vi "Set Digital IO Mode.vi"(6 "Digital IO Mode (0: IN)":enum16{"Input", "Output", "Open Drain", ""}(ring), 8 "error in (no error)":errorcluster, 9 "Digital IO Trigger Type (0: Digital)":enum16{"Digital", "Trigger"}(ring), 10 "Digital IO Line (1)":u32=1, 11 "VISA resource name":refnum<visa-resource-name>) -> (0 "error out":errorcluster, 3 "VISA resource name out":refnum<visa-resource-name>)   [LabVIEW 2020, in "Keithley 2450.lvlib"]
doc: "Sets the digital I/O line to be a digital line or trigger model line and sets the line as an input or output. You can also use this VI to configure synchronous triggering modes."
uses:
  <instrlib>/Keithley 2450/Keithley 2450.lvlib
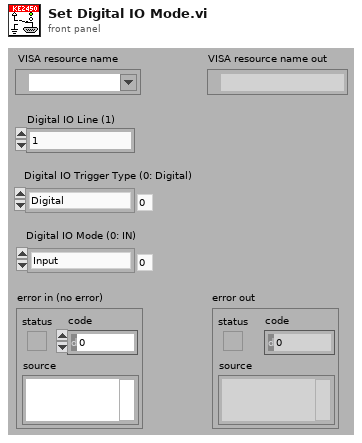
[diagram p1: front panel]
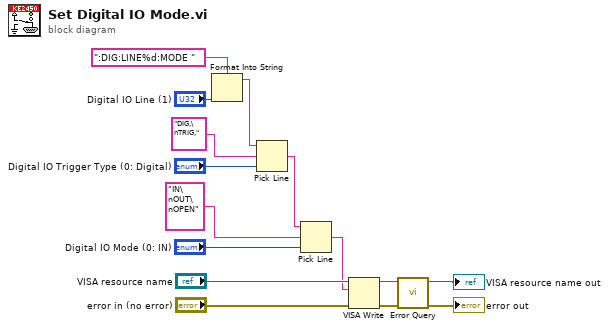
[diagram p0: block diagram]
diagram:
  n1 = Format Into String(format string=":DIG:LINE%d:MODE ", "Digital IO Line (1)") -> (resulting string=w6:string)  [unwired: 2 in, 1 out]
  n2 = Pick Line(string ("")=w6, multi-line string="DIG,\nTRIG,", line index="Digital IO Trigger Type (0: Digital)") -> (output string=w2:string)
  n3 = Pick Line(string ("")=w2, multi-line string="IN\nOUT\nOPEN", line index="Digital IO Mode (0: IN)") -> (output string=w1:string)
  n4 = VISA Write(VISA resource name="VISA resource name", write buffer=w1, error in (no error)="error in (no error)") -> (VISA resource name out=w13:refnum<visa-resource-name>, error out=w10:errorcluster)  [unwired: 1 out]
  n5 = call <instrlib>:"Error Query.vi"("error in (no error)"=w10, "VISA resource name"=w13) -> ("error out"=→"error out":errorcluster, "VISA resource name out"=→"VISA resource name out":refnum<visa-resource-name>)  [unwired: 8 out]
